vi "Populate Tree Items_TEST.vi"() -> ()   [LabVIEW 2020]
doc: "Demonstrates populating the items of the Tree control."
panel:
  in  "Third item attributes 3":string[](array[string])=["Sample 5", "Sample 6", "Sample 7", "Sample 8", "Sample 9"]
  in  "Third item attributes 2":string[](array[string])=["Sample 5", "Sample 6", "Sample 7", "Sample 8", "Sample 9"]
  in  "Active Cell:Active Column Number":i32=3
  in  "Stop Button":bool
  in  "Third item attributes":string[](array[string])=["Sample 5", "Sample 6", "Sample 7", "Sample 8", "Sample 9"]
  in  "Item indent level":i32[](array[numeric])=[0, 0, 1, 2, 3]
  in  "Second item attributes":string[](array[string])=["Sample 3", "Sample 4"]
  in  "Requested item tags":string[](array[string])=["One Tag", "Duplicate Tag", "Duplicate Tag", "Child2_Tag", "Child3_Tag"]
  in  "First item attributes":string[](array[string])=["Sample 1", "Sample 2"]
  out "Actual item tags (no duplicates)":string[](array[string])=["One Tag", "Duplicate Tag", "Duplicate Tag_1", "Child2_Tag", "Child3_Tag"]
  in  "Item names":string[](array[string])=["First item", "Duplicate", "Child1", "Child2", "Child3"]
  in  "Tree":string(tree)="Duplicate Tag_1"
  # "Overview: Demonstrates populating the items of the Tree control.\nInstructions:\n1. Run the VI to populate the Tree control.\n2. Open the block diagram for more information."
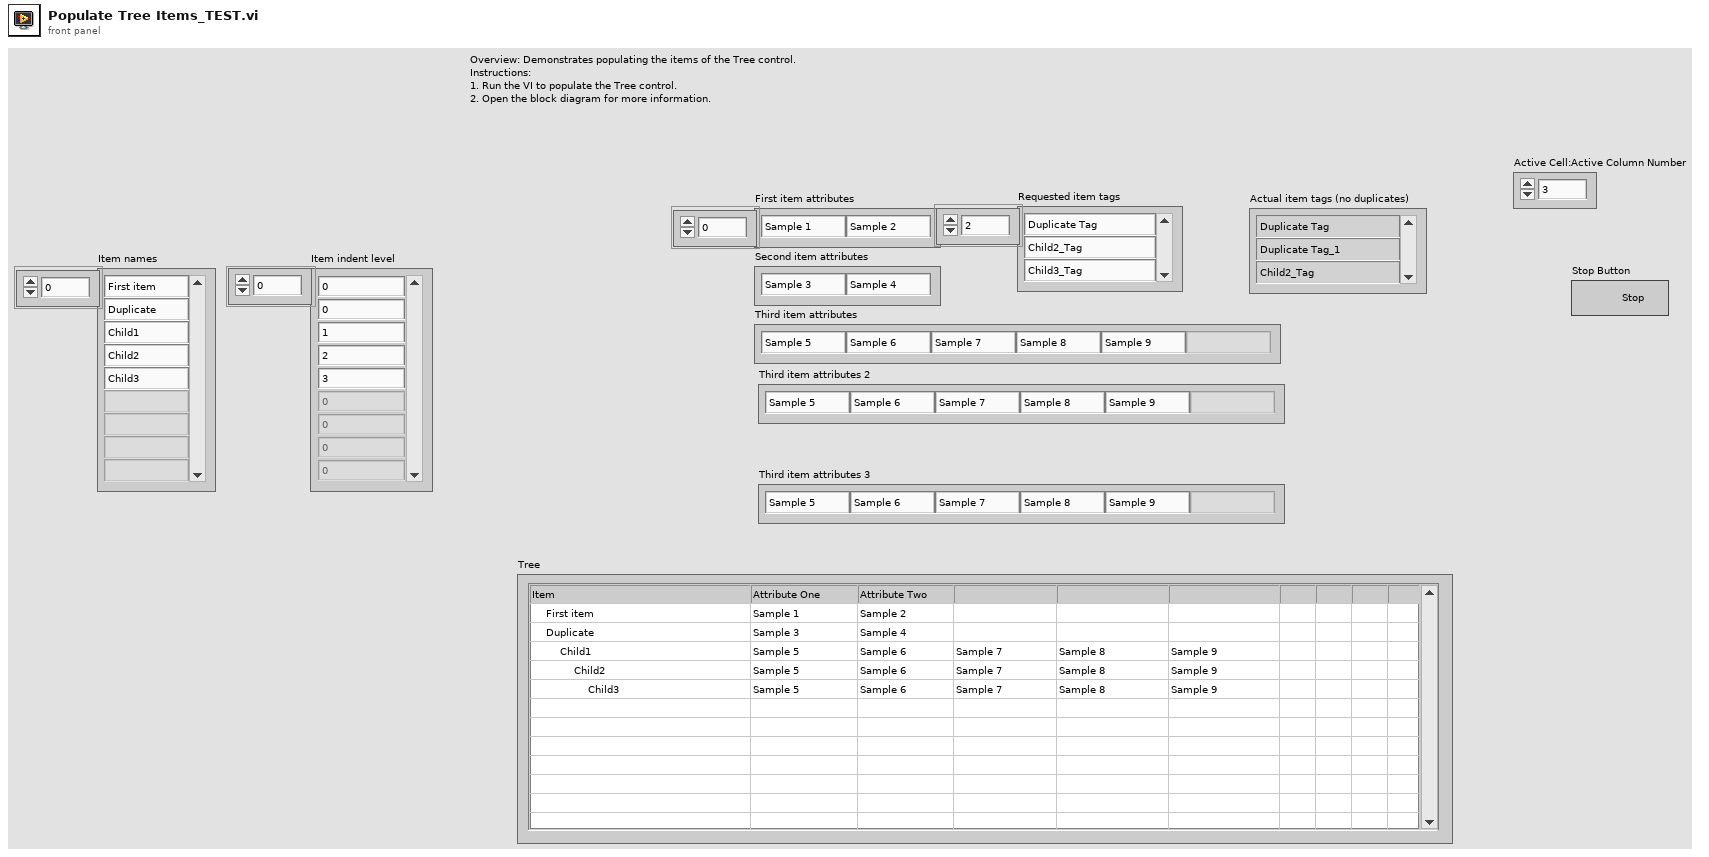
[diagram p1: front panel]
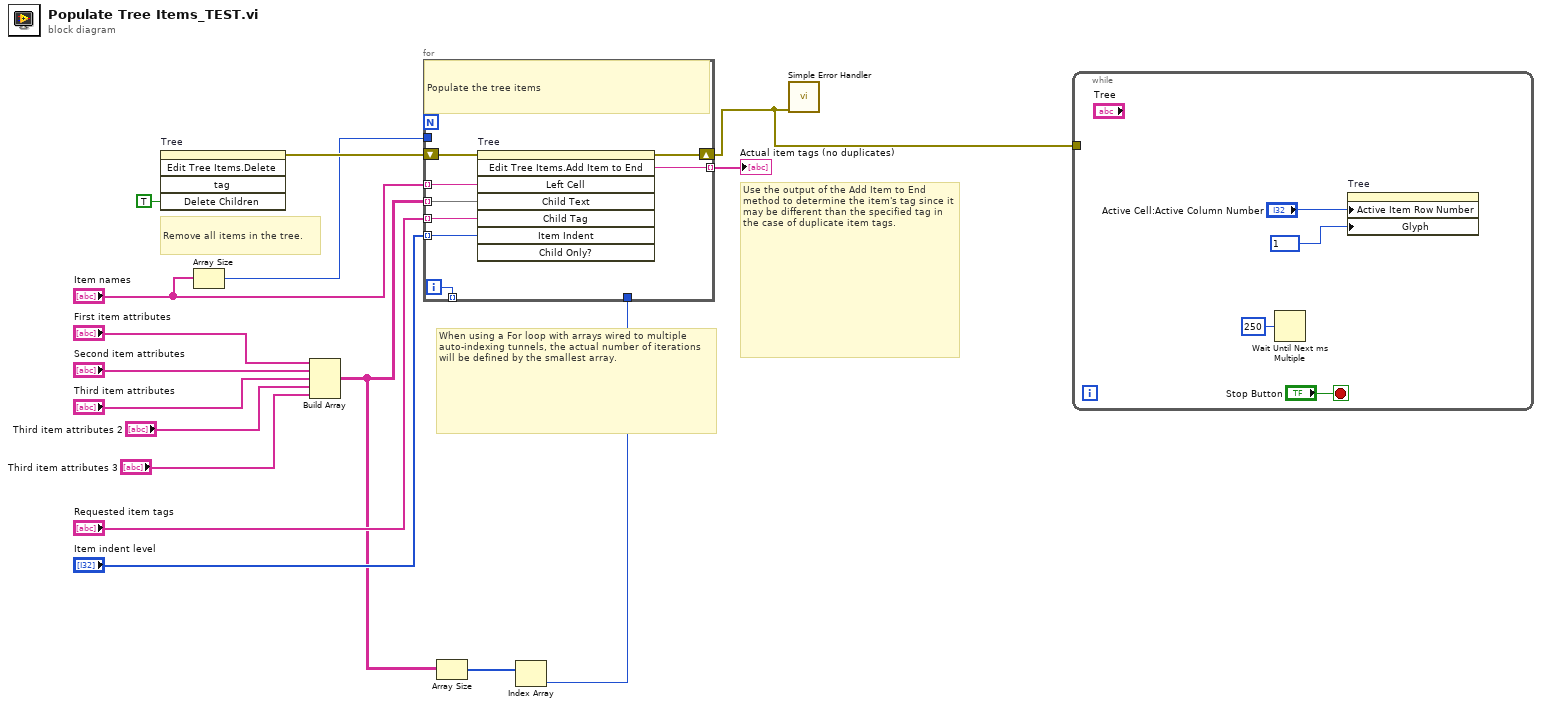
[diagram p0: block diagram]
diagram:
  # "When using a For loop with arrays wired to multiple auto-indexing tunnels, the actual number of iterations will be defined by the smallest array."
  # "Use the output of the Add Item to End method to determine the item's tag since it may be different than the specified tag in the case of duplicate item tags."
  # "Remove all items in the tree."
  n1 = invoke on="Tree" class="Tree (strict)" method="Edit Tree Items.Delete"("Delete Children"=TRUE ("Delete Children?")) -> (error out=w16:errorcluster)  [unwired: 4 in, 4 out]
  n2 = Array Size(array="Item names") -> (size(s)=w6:i32)
  n3 = Build Array("First item attributes", "Second item attributes", "Third item attributes", "Third item attributes 2", "Third item attributes 3") -> (w5:string[][])
  n4 = Array Size(array=w5) -> (size(s)=w4:i32[])
  n5 = Index Array(array=w4) -> (element=w3:i32)  [unwired: 1 in]
  n6 = for {
    tunnel: "Item names" -> [w23] mode=indexing
    tunnel: [w22] -> w15 mode=indexing
    tunnel: "Requested item tags" -> [w21] mode=indexing
    tunnel: "Item indent level" -> [w20] mode=indexing
    tunnel: w5 -> [w18] mode=indexing
    shift-right: [w19] -> w9
    shift-left: w16 -> [w24]
    tunnel: [w17] -> _ mode=indexing
    tunnel: w6 -> [_]
    tunnel: w3 -> [_]
    i -> [w17]
    # "Populate the tree items"
    n7 = invoke on="Tree" class="Tree (strict)" method="Edit Tree Items.Add Item to End"(error in=w24, "Left Cell"=w23, "Child Text"=w18, "Child Tag"=w21, "Item Indent"=w20) -> (error out=w19:errorcluster, "Edit Tree Items:Add Item to End"=w22:string)  [unwired: 3 in, 6 out]
  }
  "Actual item tags (no duplicates)" <- w15
  n8 = call <vilib>:"Simple Error Handler.vi"("error in (no error)"=w9) -> ()  [unwired: 4 in, 5 out]
  n9 = while {
    tunnel: w9 -> [_]
    stop <- "Stop Button" stop-if-true
    n10 = Wait Until Next ms Multiple(millisecond multiple=u32 250) -> ()  [unwired: 1 out]
    n11 = property on="Tree" class="Tree (strict)"("Active Item Row Number"="Active Cell:Active Column Number", "Glyph"=1) -> ()  [unwired: 2 in, 2 out]
  }
